vi "Test Gain.vi"(8 "error in (no error)":errorcluster, 11 "Instrument.Lockin in":refnum<class "Instrument.Lockin.lvclass">) -> (0 "error out":errorcluster, 3 "Instrument.Lockin out":refnum<class "Instrument.Lockin.lvclass">)   [LabVIEW 2016]
uses:
  src/Instrument.Lockin/Instrument.Lockin.lvclass
  <vilib>/addons/_JKI Toolkits/Caraya/classes/Assert/Assert Equal Value_Variant.vi
  <vilib>/addons/_JKI Toolkits/Caraya/classes/Test/Test.lvclass
  <vilib>/addons/_JKI Toolkits/Caraya/classes/Assert/Assert.lvclass
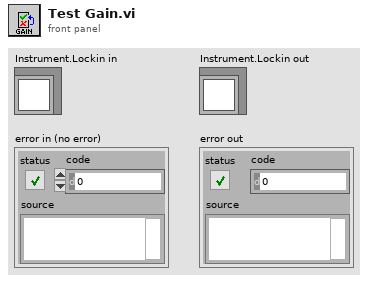
[diagram p1: front panel]
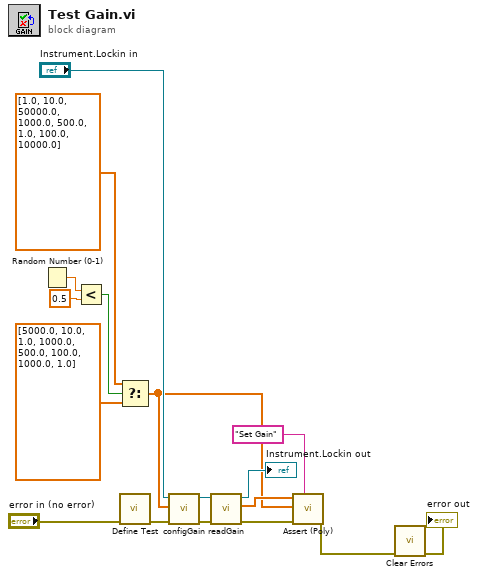
[diagram p0: block diagram]
diagram:
  n1 = Random Number (0-1)() -> (number: 0 to 1=w10:dbl)
  n2 = Less?(x=w10, y=0.5) -> (x < y?=w7:bool)
  n3 = Select(t=dbl[] [1.0, 10.0, 50000.0, 1000.0, 500.0, 1.0, 100.0, 10000.0] ("Gain"), s=w7, f=dbl[] [5000.0, 10.0, 1.0, 1000.0, 500.0, 100.0, 1000.0, 1.0] ("Gain")) -> (s? t:f=w5:dbl[])
  n4 = call <vilib>:"Define Test.vi"("error in (no error)"="error in (no error)") -> ("error out"=w17:errorcluster)  [unwired: 10 in]
  n5 = call "configGain.vi"("error in (no error)"=w17, "Gain"=w5, "Instrument.Lockin in"="Instrument.Lockin in") -> ("error out"=w14:errorcluster, "Instrument.Lockin out"=w13:refnum<class "Instrument.Lockin.lvclass">)  [unwired: 7 in]
  n6 = call "readGain.vi"("error in (no error)"=w14, "Instrument.Lockin in"=w13) -> ("error out"=w4:errorcluster, "Gain"=w11:dbl[], "Instrument.Lockin out"=→"Instrument.Lockin out":refnum<class "Instrument.Lockin.lvclass">)  [unwired: 7 in]
  n7 = call-poly <vilib>:"Assert (Poly).vi"("Label"="Set Gain", "error in (no error)"=w4, "Y"=w5, "X"=w11) -> ("error out"=w2:errorcluster)  [unwired: 7 in]
  n8 = call <vilib>:"Clear Errors.vi"("error in (no error)"=w2) -> ("error out"=→"error out":errorcluster)  [unwired: 5 in, 1 out]
